vi "test_LoadCommandlineArgs_LogFile.vi"() -> (3 "Pass?":bool)   [LabVIEW 2019, in "Tests.SolutionBuilder.lvlib"]
uses:
  Tests.SolutionBuilder.lvlib
  SolutionBuilder/SolutionBuilder.lvclass
  SolutionBuilder/Community/Options.ctl
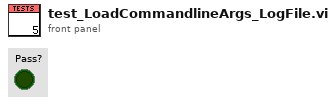
[diagram p1: front panel]
types:
  T1 = typedef "SolutionBuilder.lvlib/SolutionBuilder.lvclass/Options.ctl" = cluster{"Path":path, "Preview?":bool, "Quiet?":bool, "Log file":path, "Success file":path, "Rebuild?":bool, "Keep split projects?":bool}
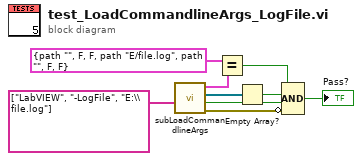
[diagram p0: block diagram]
diagram:
  n1 = call "subLoadCommandlineArgs.vi"("App.Args"=string[] ["LabVIEW", "-LogFile", "E:\\file.log"]) -> ("error out"=w2:errorcluster, "From command line?"=w8:bool, "Pre-built libraries"=w5:refnum<class "ProjectItem.lvclass">[], "Options"=w4:T1)  [unwired: 6 in, 1 out]
  n2 = Equal?(x=T1 {"Path"=path "", "Preview?"=FALSE, "Quiet?"=FALSE, "Log file"=path "E:/file.log", "Success file"=path "", "Rebuild?"=FALSE, "Keep split projects?"=FALSE} ("Options"), y=w4) -> (x = y?=w7:bool)
  n3 = Empty Array?(array=w5) -> (empty?=w6:bool)
  n4 = Compound Arithmetic op=AND(w7, w6, w8, invert w2) -> (→"Pass?":bool)
